vi "animal_drawer.vi"() -> ()   [LabVIEW 2024]
panel:
  out "appended array":dbl[](array[numeric])
  out "2D Picture 2":picture
  in  "end effector":cluster{dbl, dbl}={159.01647214211073, 1.9100783062530127} {"?" format="%.1f"; "?" format="%#.1f"}
  out "Angle1":dbl(knob)=-45.83837436417874 scale=-90.0..90.0
  out "Angle 2":dbl(knob)=-72.06882847083946 scale=-90.0..90.0
  in  "L 1":dbl(slide)=80.0 scale=0.0..200.0
  in  "L 2":dbl(slide)=115.0 scale=0.0..200.0
  out "2D Picture":picture
  out "end effector 2":cluster{dbl, dbl}={159.01647214211073, 1.9100783062530127} {"?" format="%.1f"; "?" format="%#.1f"}
  in  "?":bool
  out "initialized array":cluster{dbl, dbl}[](array[cluster])
  # "mm"
  # "mm"
  # "mm"
  # "mm"
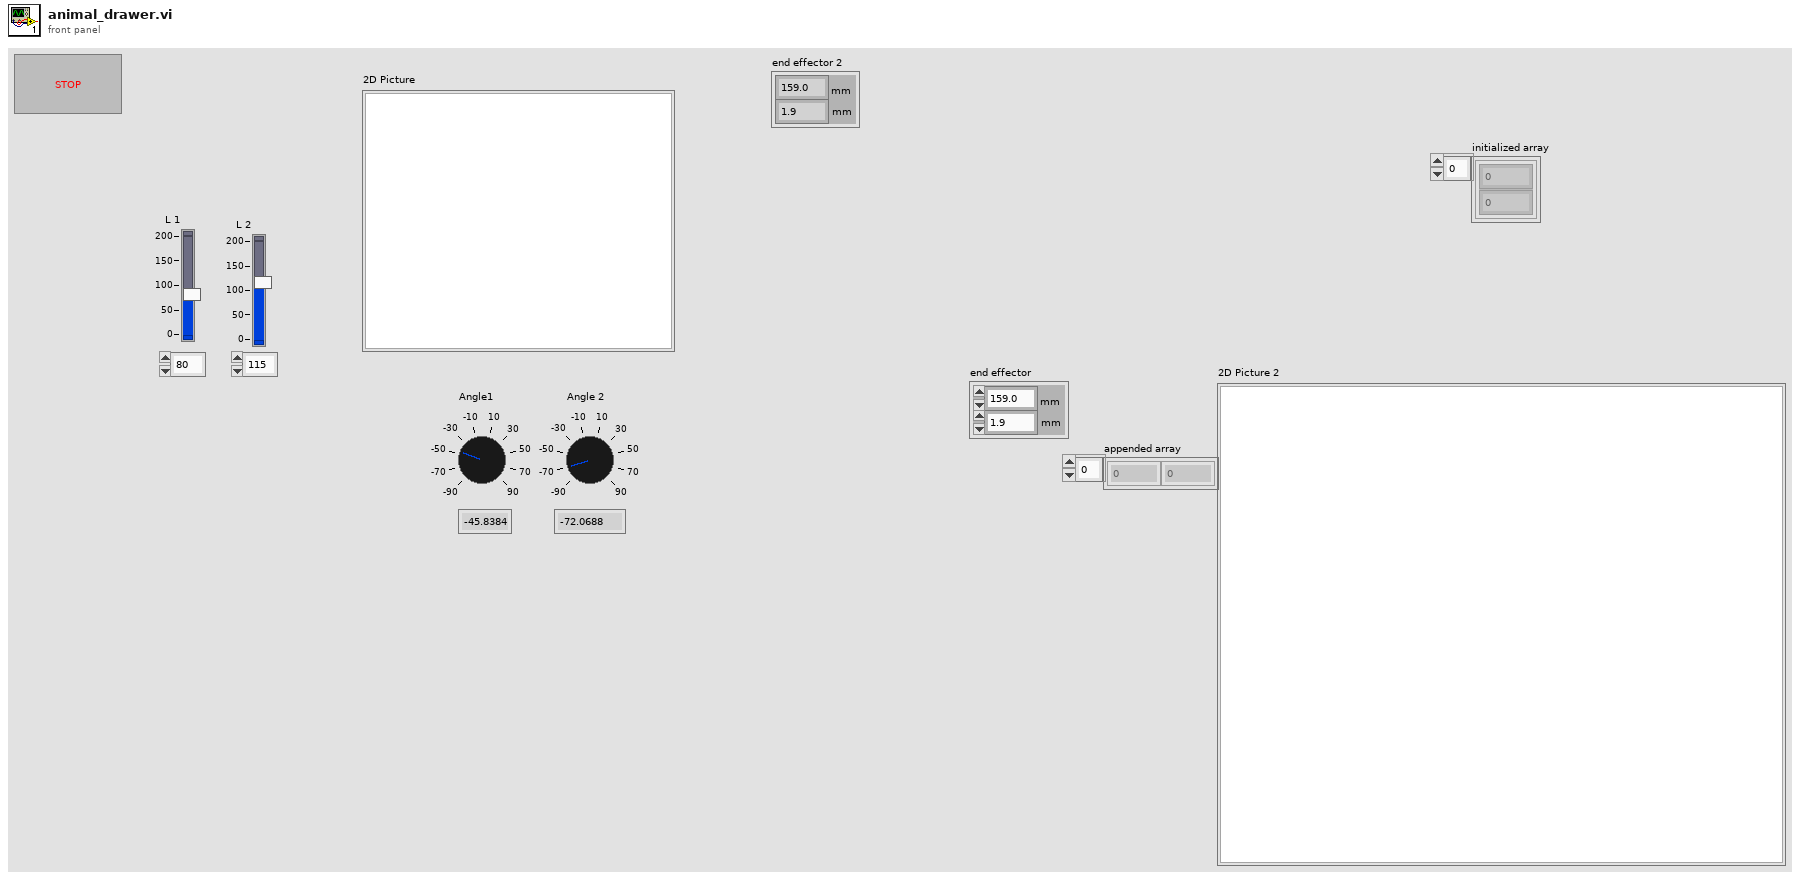
[diagram p1: front panel]
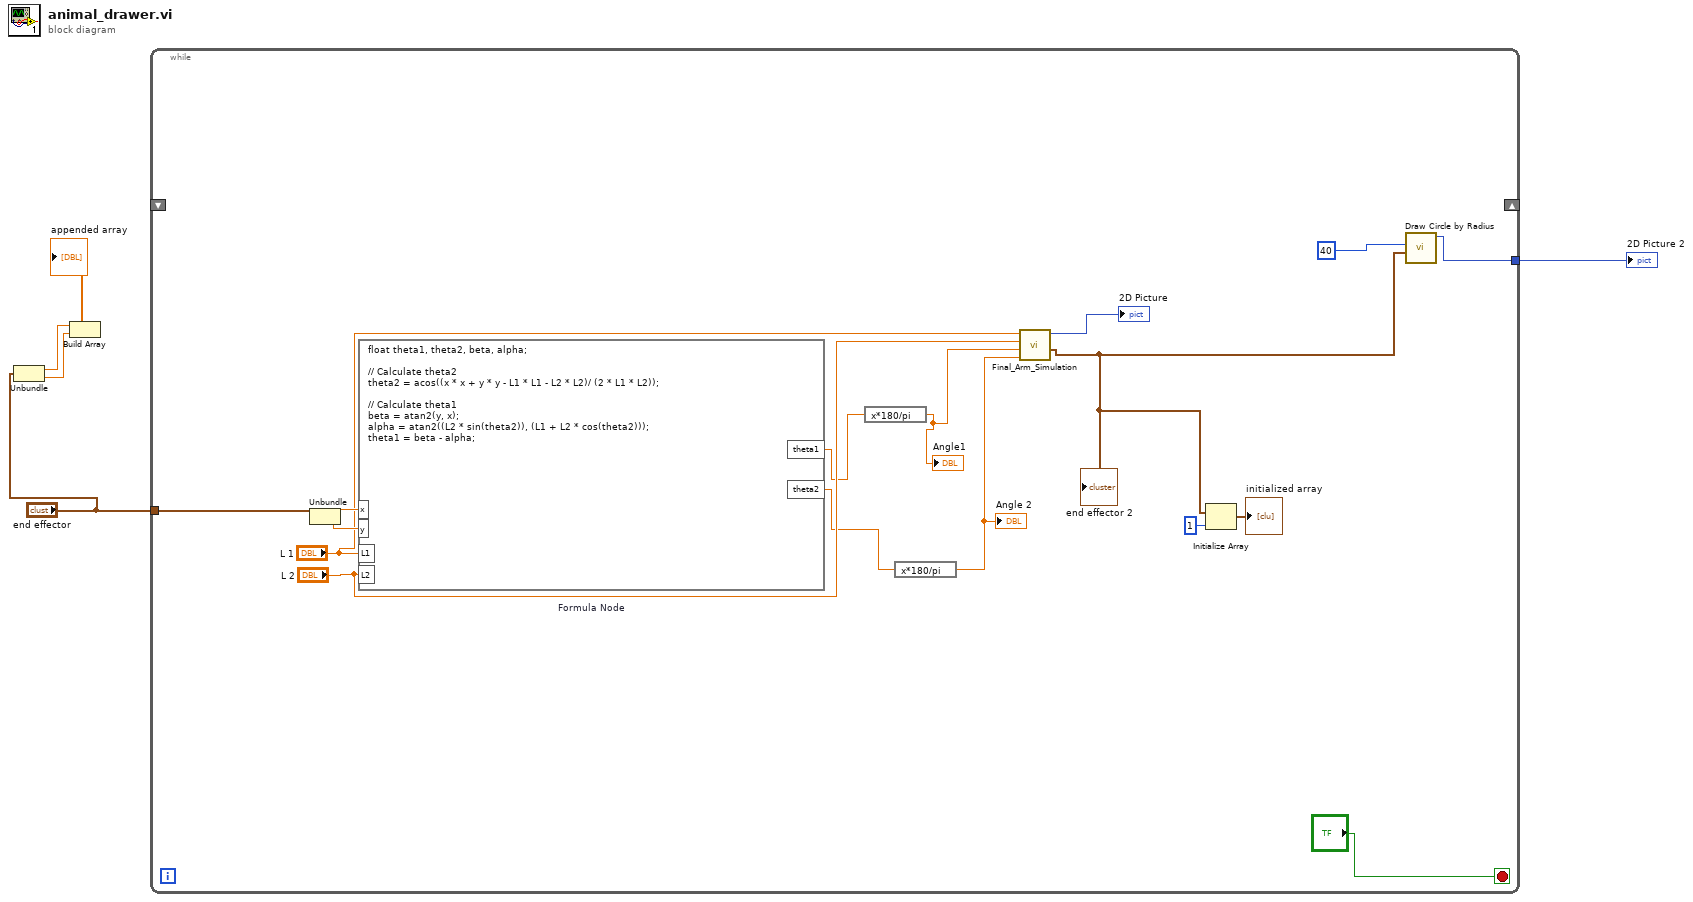
[diagram p0: block diagram]
diagram:
  n1 = Unbundle("end effector") -> (w3:dbl, w2:dbl)
  n2 = Build Array(w3, w2) -> (→"appended array":dbl[])
  n3 = while {
    tunnel: "end effector" -> [w8]
    shift-right: _ -> [_]
    shift-left: _ -> [_]
    tunnel: [w6] -> w1
    stop <- "?" stop-if-true
    n4 = Unbundle(w8) -> (w21:dbl, w20:dbl)
    n5 = formula code="float theta1, theta2, beta, alpha;\n\n// Calculate theta2\ntheta2 = acos((x * x + y * y - L1 * L1 - L2 * L2)/ (2 * L1 * L2));\n\n// Calculate theta1\nbeta = atan2(y, x);\nalpha = atan2((L2 * sin(theta2)), (L1 + L2 * cos(theta2)));\ntheta1 = beta - alpha;"("L1"="L 1", "L2"="L 2", "x"=w21, "y"=w20) -> ("theta1"=w13:dbl, "theta2"=w16:dbl)
    n6 = expression code="x*180/pi"(w13) -> (w14:dbl)
    "Angle1" <- w14
    n7 = expression code="x*180/pi"(w16) -> (w15:dbl)
    "Angle 2" <- w15
    n8 = call "Final_Arm_Simulation.vi"("Angle 2"=w15, "Angle1"=w14, "L 2"="L 2", "L 1"="L 1") -> ("end effector"=w11:cluster{dbl, dbl}, "2D Picture"=→"2D Picture":picture)  [unwired: 6 in]
    "end effector 2" <- w11
    n9 = Initialize Array(w11, 1 ("dimension size")) -> (→"initialized array":cluster{dbl, dbl}[])
    n10 = call <vilib>:"Draw Circle by Radius.vi"("pixel center"=w11, "radius"=i16 40) -> ("new picture"=w6:picture)  [unwired: 9 in]
  }
  "2D Picture 2" <- w1
